vi "Update All.vi"(0 "reference in":refnum<class "DO.lvclass">, 5 "error in (no error)":errorcluster) -> (14 "reference out":refnum<class "DO.lvclass">, 19 "error out":errorcluster)   [LabVIEW 2017, in "DO.lvclass"]
uses:
  DO.lvclass
  <vilib>/DAQmx/write.llb/DAQmx Write (Digital 1D Bool NChan 1Samp 1Line).vi
  <vilib>/DAQmx/miscellaneous.llb/DAQmx Fill In Error Info.vi
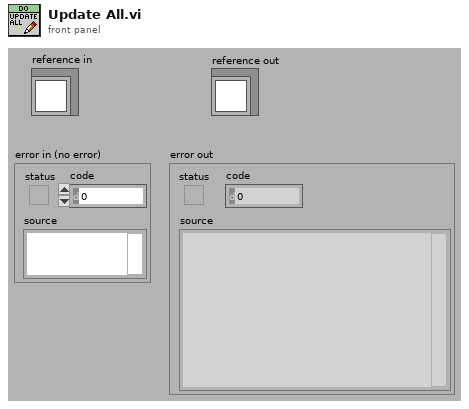
[diagram p1: front panel]
types:
  T1 = typedef "DO.lvclass/ObjectAttributes.ctl" = cluster{"DO Task":refnum<k21>, "DO Module Names (NI-Max Name)":string[], "Number of Channels Per DO Module":i32[], "DO Status":bool[], "Number of DO Modules":u32, "DO Status to Set":bool[], "DO On/Off Status":bool, "DO VI Reference":refnum<vi>, "Number of Total DO Channels":u32}
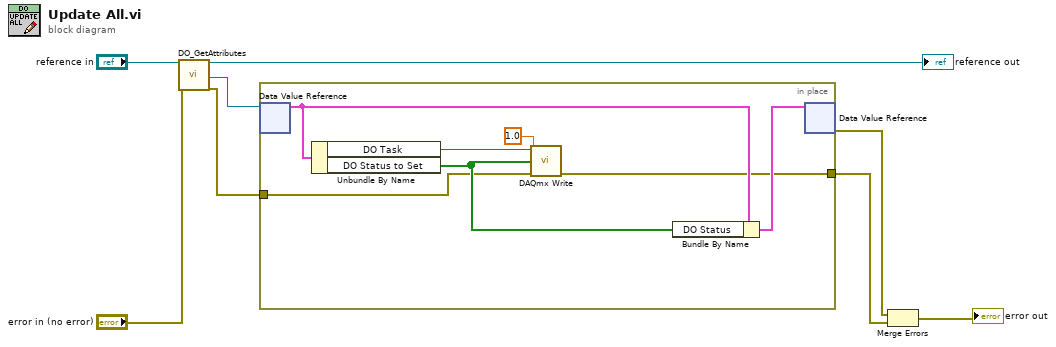
[diagram p0: block diagram]
diagram:
  n1 = call "DO_GetAttributes.vi"("reference in"="reference in", "error in (no error)"="error in (no error)") -> ("reference out"=→"reference out":refnum<class "DO.lvclass">, "DataRef"=w3:refnum<data-value>, "error out"=w2:errorcluster)  [unwired: 14 in, 1 out]
  n2 = in-place {
    in-place-border: w2 -> [w10]
    in-place-border: [w12] -> w1
    n3 = in-place-dvr #1(w3) -> (w14:T1)  [unwired: 1 out]
    n4 = Unbundle By Name(w14) -> ("DO Task"=w11:refnum<k21>, "DO Status to Set"=w13:bool[])
    n5 = call-poly <vilib>:"DAQmx Write.vi"("task/channels in"=w11, "data"=w13, "timeout"=1.0, "error in"=w10) -> ("error out"=w12:errorcluster)  [unwired: 9 in, 2 out]
    n6 = Bundle By Name(cluster=w14, "DO Status"=w13) -> (w15:T1)
    n7 = in-place-dvr #1(w15) -> (w4:errorcluster)  [unwired: 1 out]
  }
  n8 = Merge Errors(w4, w1) -> (→"error out":errorcluster)
